vi "Test Webcam.vi"() -> ()   [LabVIEW 2011]
uses:
  <vilib>/vision/NI_Vision_Development_Module.lvlib
panel:
  in  "Camera Data":T1={"Pan::Mode"=2, "Pan::Value"=0, "Tilt::Mode"=2, "Tilt::Value"=0, "Number of Image Buffers"=10, "Stop (F)"=FALSE, "Zoom::Mode"=2, "Zoom::Value"=0} {"Zoom::Value" min=0 max=10 step=1; "Zoom::Mode" items=["Manual"=2]; "Tilt::Value" min=-10 max=10 step=1; "Tilt::Mode" items=["Manual"=2]; "Pan::Value" min=-10 max=10 step=1; "Pan::Mode" items=["Manual"=2]}
  out "Altered Image":T2(plugin-control)
  in  "Stop Button":bool
  in  "Replace Blue With":enum16{"Red", "Green", "Blue"}(ring)
  in  "Replace Green With":enum16{"Red", "Green", "Blue"}(ring)=enum."Blue"
  in  "Replace Red With":enum16{"Red", "Green", "Blue"}(ring)=enum."Green"
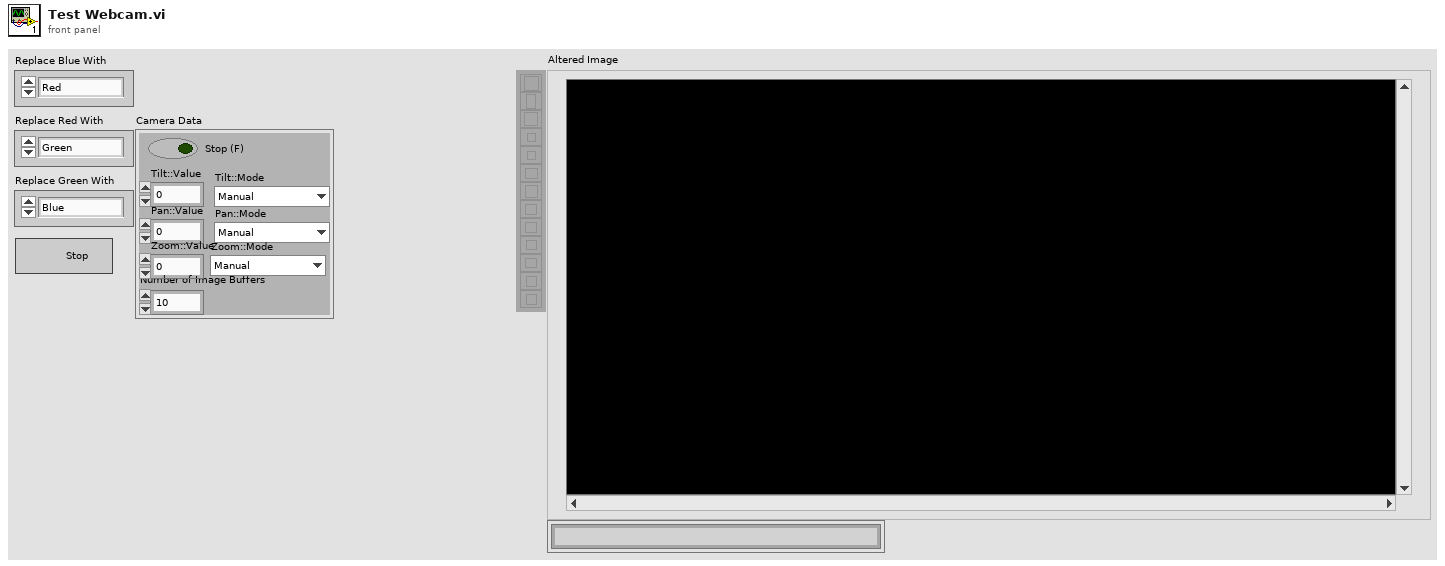
[diagram p1: front panel]
types:
  T1 = cluster{"Pan::Mode":u32, "Pan::Value":i64, "Tilt::Mode":u32, "Tilt::Value":i64, "Number of Image Buffers":u32, "Stop (F)":bool, "Zoom::Mode":u32, "Zoom::Value":i64}
  T2 = typedef "IMAQ Image.ctl" = refnum<image>
  T3 = typedef "Image Type" = u32
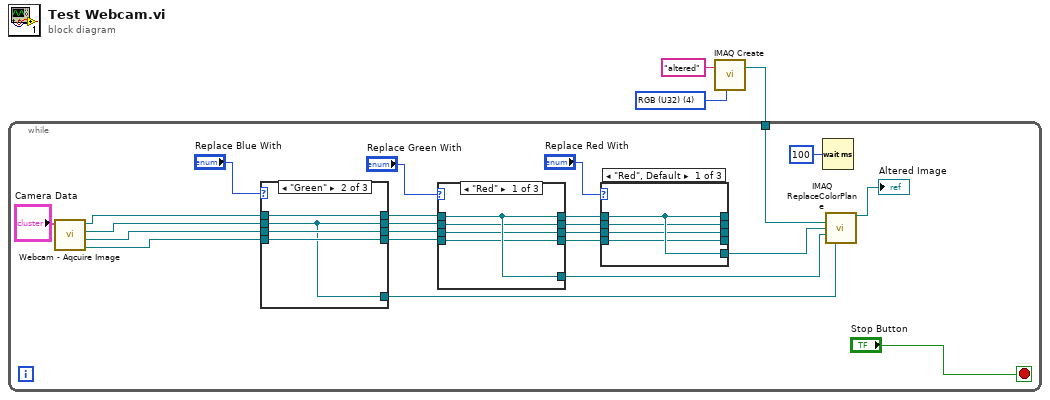
[diagram p0: block diagram]
diagram:
  w3 = T3 4 items=["Grayscale (U8)", "Grayscale (I16)", "Grayscale (SGL)", "Complex (CSG)", "RGB (U32)", "HSL (U32)", "RGB (U64)", "Grayscale (U16)"] ("Image Type")
  n1 = call "IMAQ Create"("Image Name"="altered", "Image Type"=w3) -> ("New Image"=w1:T2)  [unwired: 3 in, 1 out]
  n2 = while {
    tunnel: w1 -> [w26]
    stop <- "Stop Button" stop-if-true
    n3 = call "Webcam - Aqcuire Image.vi"("Camera Data"="Camera Data") -> ("Blue or Luma or Val or Inten Plane out"=w22:T2, "Green or Sat Plane out"=w23:T2, "Red or Hue Plane out"=w24:T2, "Webcam Out"=w25:T2)  [unwired: 7 in]
    n4 = case shown="\"Green\"" "Replace Blue With" {
      tunnel: w25 -> [w54 w57 w62]
      tunnel: w24 -> [w53 w55 w61]
      tunnel: w23 -> [w52 w56 w59]
      tunnel: w22 -> [w51 w58 w60]
      tunnel: [w51 w58 w60] -> w18
      tunnel: [w54 w57 w62] -> w21
      tunnel: [w53 w55 w61] -> w20
      tunnel: [w52 w56 w59] -> w19
      tunnel: [w54 w55 w59] -> w11
      frame "Red" {
      }
      frame "Green" {
      }
      frame "Blue", Default {
      }
    }
    n5 = case shown="\"Red\"" "Replace Green With" {
      tunnel: w21 -> [w42 w45 w50]
      tunnel: w20 -> [w41 w43 w49]
      tunnel: w19 -> [w40 w44 w47]
      tunnel: w18 -> [w39 w46 w48]
      tunnel: [w39 w46 w48] -> w14
      tunnel: [w42 w45 w50] -> w17
      tunnel: [w41 w43 w49] -> w16
      tunnel: [w40 w44 w47] -> w15
      tunnel: [w42 w43 w47] -> w12
      frame "Red" {
      }
      frame "Green", Default {
      }
      frame "Blue" {
      }
    }
    n6 = case shown="\"Red\", Default" "Replace Red With" {
      tunnel: w17 -> [w30 w33 w38]
      tunnel: w16 -> [w29 w31 w37]
      tunnel: w15 -> [w28 w32 w35]
      tunnel: w14 -> [w27 w34 w36]
      tunnel: [w27 w34 w36] -> _
      tunnel: [w30 w33 w38] -> _
      tunnel: [w29 w31 w37] -> _
      tunnel: [w28 w32 w35] -> _
      tunnel: [w30 w31 w35] -> w13
      frame "Red", Default {
      }
      frame "Green" {
      }
      frame "Blue" {
      }
    }
    n7 = Wait (ms)(milliseconds to wait=u32 100) -> ()  [unwired: 1 out]
    n8 = call "IMAQ ReplaceColorPlane"("Image Dst"=w26, "Red or Hue Plane"=w13, "Green or Sat Plane"=w12, "Blue or Luma or Val or Inten Plane"=w11) -> ("Image Dst Out"=→"Altered Image":T2)  [unwired: 10 in, 1 out]
  }
